vi "build auth URI.vi"(8 "error in (no error)":errorcluster, 10 "State Parameter":string, 11 "Oauth2.Google in":refnum<class "Oauth2.Google.lvclass">) -> (0 "error out":errorcluster, 2 "Authorization Request URI":string, 3 "Oauth2":refnum<class "Oauth2.lvclass">)   [LabVIEW 2017, in "Oauth2.Google.lvclass"]
uses:
  Oauth2.Google.lvclass
  D:/GitHub/Oauth2/source/Oauth2/Oauth2.lvclass
  Oauth2/Oauth2.lvclass
  OAuthToken/OAuth2 Token Element -- enum.ctl
  LabVIEW/Oauth2/source/Oauth2/OAuth2 Response Type -- ring.ctl
  OAuthToken/OAuthAccessToken.lvclass
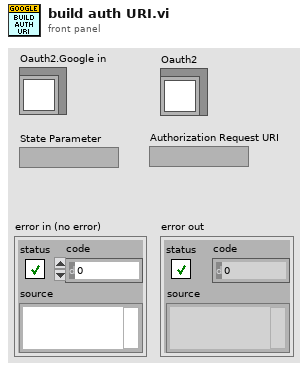
[diagram p1: front panel]
types:
  T1 = typedef "Oauth2.lvclass/OAuth2 Response Type -- ring.ctl" = string
  T2 = typedef "OAuthAccessToken.lvclass/OAuth2 Token Element -- enum.ctl" = enum16{"client_id", "client_secret", "response_type", "scope", "redirect_uri", "error", "error_description", "error_uri", "grant_type", "code", "access_token", "token_type", "expires_in", "username", "password", "refresh_token", "code_challenge", "code_challenge_method", "reverse_proxy_uri", "endpoint element", "access_type", "prompt", "id_token"}
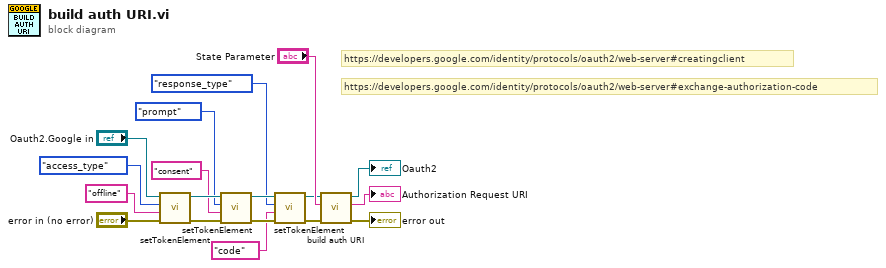
[diagram p0: block diagram]
diagram:
  # "https://developers.google.com/identity/protocols/oauth2/web-server#exchange-authorization-code"
  # "https://developers.google.com/identity/protocols/oauth2/web-server#creatingclient"
  n1 = call "setTokenElement.vi"("error in (no error)"="error in (no error)", "Value"="offline", "Token element"=OAuth2_Token_Element_--_enum."access_type", "Oauth2 in"="Oauth2.Google in") -> ("error out"=w11:errorcluster, "Oauth2 out"=w10:refnum<class "Oauth2.Google.lvclass">)  [unwired: 6 in]
  n2 = call "setTokenElement.vi"("error in (no error)"=w11, "Value"="consent", "Token element"=OAuth2_Token_Element_--_enum."prompt", "Oauth2 in"=w10) -> ("error out"=w5:errorcluster, "Oauth2 out"=w6:refnum<class "Oauth2.Google.lvclass">)  [unwired: 6 in]
  n3 = call "setTokenElement.vi"("error in (no error)"=w5, "Value"=T1 "code", "Token element"=OAuth2_Token_Element_--_enum."response_type", "Oauth2 in"=w6) -> ("error out"=w1:errorcluster, "Oauth2 out"=w2:refnum<class "Oauth2.Google.lvclass">)  [unwired: 6 in]
  n4 = call-parent "build auth URI.vi"("error in (no error)"=w1, "State Parameter"="State Parameter", "Oauth2 in"=w2) -> ("error out"=→"error out":errorcluster, "Authorization Request URI"=→"Authorization Request URI":string, "Oauth2"=→"Oauth2":refnum<class "Oauth2.lvclass">)  [unwired: 6 in]
